vi "ShapeDetect_Setting_UI.vi"(8 "error in (no error)":errorcluster, 10 "ParameterIn":string, 11 "Vision_Image":T8(plugin-control)) -> (0 "error out":errorcluster, 1 "Cancel?":bool, 3 "ParameterOut":string)   [LabVIEW 2019]
uses:
  Controls/_UI Command Cluster/ShapeDetect_UICommand.ctl
  <vilib>/Utility/miscctls.llb/LVPointTypeDef.ctl
  Controls/V_Analysis_Type.ctl
  Controls/ShapeDectect/Analysis_ShapeDectect_Parameter.ctl
  Controls/Analysis_Setting.ctl
  <vilib>/vision/Image Controls.llb/IMAQ Image.ctl
  bd2e2234-6d1e-4fcc-8dd9-21a115e7fd9b.vi
  bb507319-f4b5-469f-81a6-a6debf547fbf.vi
  52026581-d36c-43e1-9bb6-5096a44cea8b.vi
  <vilib>/JDP Science/JSONtext/JSON text to Variant.vi
  <vilib>/JDP Science/JSONtext/Variant to JSON Text.vi
  <vilib>/vision/NI_Vision_Development_Module.lvlib
panel:
  in  "Show Curve":bool
  out "Message":string
  in  "Tab":enum32{"Curve", "Shape", "Setting", "Result"}(tab)
  in  "Curve Extraction":T1={"Extraction Mode"=0, "Edge Threshold"=75, "Edge Filter Size"=1, "Min Length"=25, "Row Search Step Size"=15, "Column Search Step Size"=15, "Max Endpoint Gap"=10, "Closed"=FALSE, "Subpixel"=FALSE} {"Edge Filter Size" items=["Fine", "Normal", "Contour Tracing"]; "Edge Threshold" min=0 max=255 step=1; "Extraction Mode" items=["Normal", "Uniform Regions"]}
  in  "Shape Type":T2(ring)
  out "DecriptroTab":T3(tab)
  in  "Circle Descriptor":T4={"Min Radius"=10.0, "Max Radius"=100.0, "Min"=10.0, "Max"=100.0} {"Max" min=10.0 max=100.0 step=1.0; "Min" min=3.0 max=10.0 step=1.0; "Min Radius" min=3.0 max=200.0 step=1.0; "Max Radius" min=10.0 step=1.0}
  in  "Ellipse Descriptor":T5={"Min Major Radius"=10.0, "Max Major Radius"=100.0, "Min Minor Radius"=10.0, "Max Minor Radius"=100.0} {"Max Major Radius" min=10.0 max=5000.0; "Min Major Radius" min=3.0 max=100.0 step=1.0; "Min Minor Radius" min=3.0 max=100.0 step=1.0; "Max Minor Radius" min=10.0 max=5000.0 step=1.0}
  in  "Line Descriptor":T6={"Min Length"=10.0, "Max Length"=100.0, "Min"=10.0, "Max"=100.0} {"Max" min=3.0 step=1.0; "Min" min=3.0 step=1.0; "Min Length" min=3.0 max=100.0 step=1.0; "Max Length" min=10.0 step=1.0}
  in  "Rectangle Descriptor":T7={"Min Height"=10.0, "Max Height"=100.0, "Min Width"=10.0, "Max Width"=100.0} {"Max Width" min=10.0 max=5000.0 step=1.0; "Min Width" min=3.0 max=100.0 step=1.0; "Min Height" min=3.0 max=100.0 step=1.0; "Max Height" min=10.0 max=5000.0 step=1.0}
  in  "Score":dbl=800.0 min=0.0 max=1000.0 step=1.0
  in  "Number to Detect":i32=1 min=1 step=1
  out "Result":string[][](table)
  in  "ReadImage":bool
  in  "Cancel":bool
  in  "OK":bool
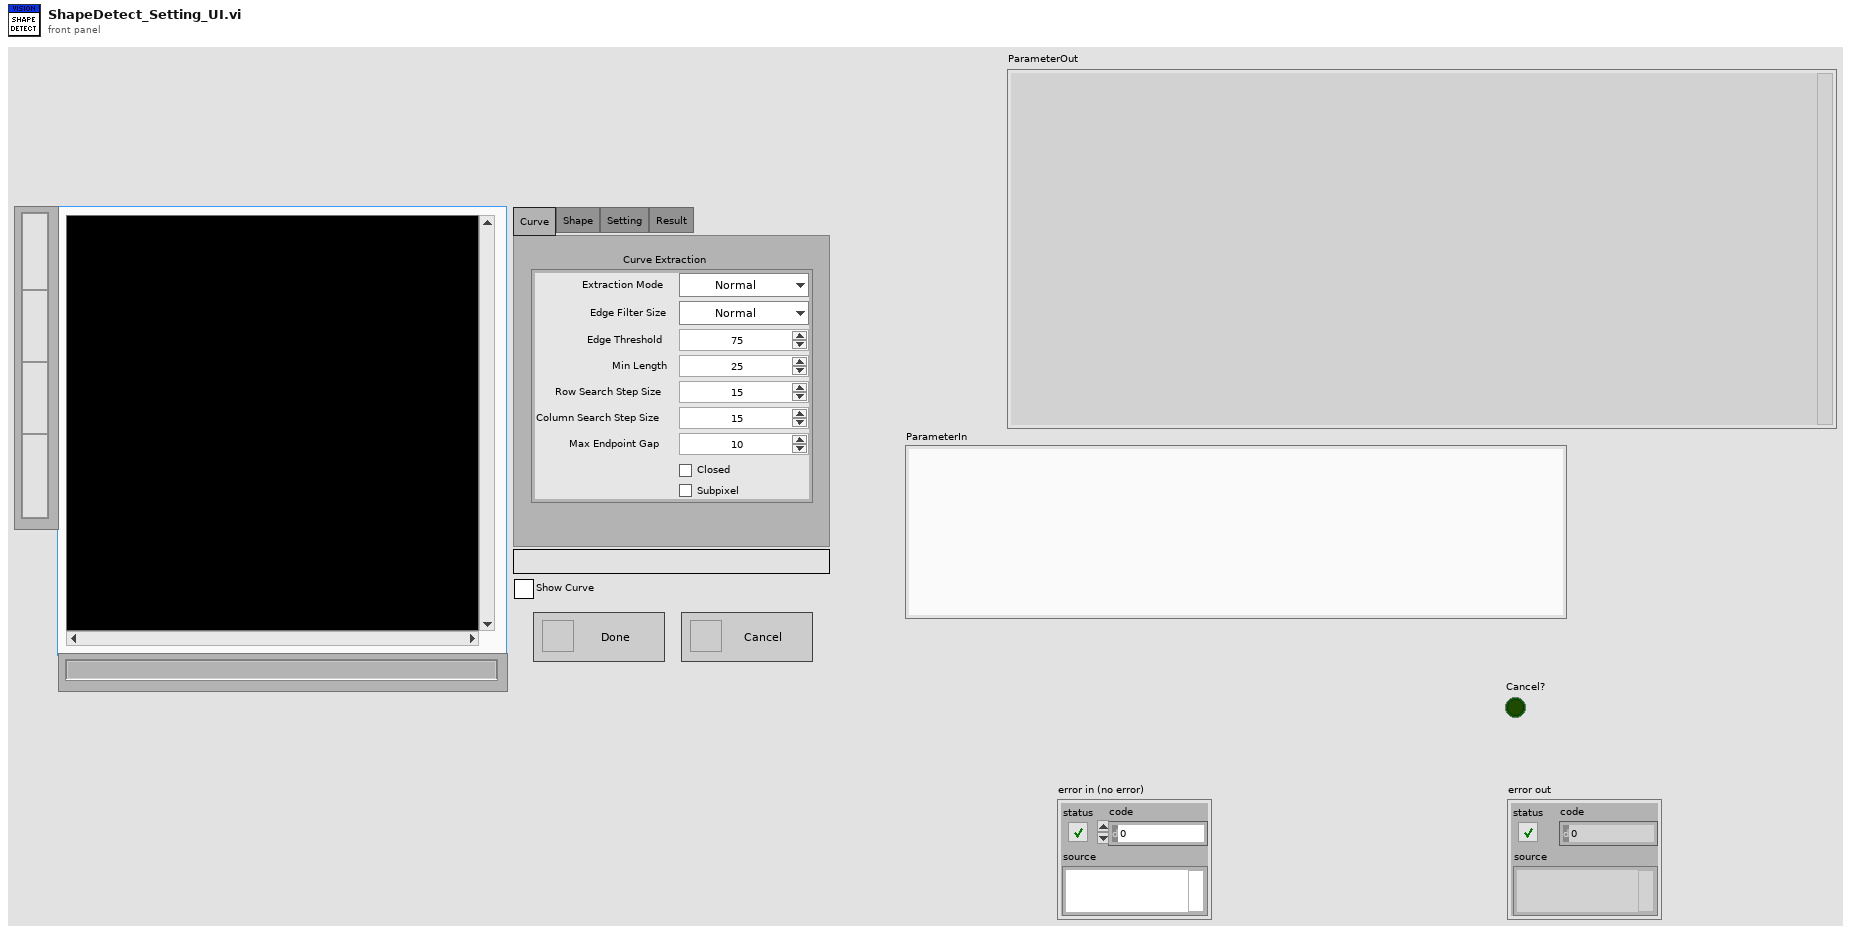
[diagram p1: front panel]
types:
  T1 = cluster{"Extraction Mode":u32, "Edge Threshold":i32, "Edge Filter Size":u32, "Min Length":i32, "Row Search Step Size":i32, "Column Search Step Size":i32, "Max Endpoint Gap":i32, "Closed":bool, "Subpixel":bool}
  T2 = enum16{"Circles", "Ellipses", "Lines", "Rectangles"}
  T3 = enum32{"Circles", "Ellipses", "Lines", "Rectangles"}
  T4 = cluster{"Min Radius":dbl, "Max Radius":dbl, "Min":dbl, "Max":dbl}
  T5 = cluster{"Min Major Radius":dbl, "Max Major Radius":dbl, "Min Minor Radius":dbl, "Max Minor Radius":dbl}
  T6 = cluster{"Min Length":dbl, "Max Length":dbl, "Min":dbl, "Max":dbl}
  T7 = cluster{"Min Height":dbl, "Max Height":dbl, "Min Width":dbl, "Max Width":dbl}
  T8 = typedef "IMAQ Image.ctl" = refnum<image>
  T9 = typedef "LVPointTypeDef.ctl" = cluster{"Horizontal":i16, "Vertical":i16}
  T10 = typedef "ShapeDetect_UICommand.ctl" = cluster{"Message":enum16{"Initialize", "InitializeUI", "CheckDescriptor", "RunAlgorithm", "Done", "Cancel", "Exit"}, "Data":variant}
  T11 = typedef "V_Analysis_Type.ctl" = enum16{"None", "C_Color Pattern Matching", "G_PatternMatching", "G_ShapeDectect", "G_GeometricMatch", "B_Area Check"}
  T12 = typedef "Analysis_ShapeDectect_Parameter.ctl" = cluster{"Enum_ShapeType":enum16{"Circles", "Ellipses", "Lines", "Rectangles"}, "MaxParticle":i32, "Descriptor":cluster{"Set 1":dbl, "Set 2":dbl, "Set 3":dbl, "Set 4":dbl}, "Match Options":cluster{"Rotation":bool, "Scale":bool, "Occlusion":bool, "Range Settings":cluster{"Match Constraints":u32, "Min":dbl, "Max":dbl}[]}, "Curve Parameters":cluster{"Extraction Mode":u32, "Edge Threshold":i32, "Edge Filter Size":u32, "Min Length":i32, "Row Search Step Size":i32, "Col Search Step Size":i32, "Max Endpoint Gap":i32, "Closed":bool, "Subpixel":bool}, " score":dbl}
  T13 = cluster{"Rotation":bool, "Scale":bool, "Occlusion":bool, "Range Settings":cluster{"Match Constraints":u32, "Min":dbl, "Max":dbl}[]}
  T14 = cluster{"Global Rectangle":i32[], "Contours":cluster{"ID":enum32{"External", "Internal"}, "Type":u32, "Coordinates":i32[]}[]}
  T15 = typedef "Analysis_Setting.ctl" = cluster{"PreProcess":T11, "Parameter":string}
  T16 = enum16{"Initialize", "InitializeUI", "CheckDescriptor", "RunAlgorithm", "Done", "Cancel", "Exit"}
  T17 = typedef "Image Type" = u32
  T18 = cluster{"Set 1":dbl, "Set 2":dbl, "Set 3":dbl, "Set 4":dbl}
  T19 = cluster{"Extraction Mode":u32, "Edge Threshold":i32, "Edge Filter Size":u32, "Min Length":i32, "Row Search Step Size":i32, "Col Search Step Size":i32, "Max Endpoint Gap":i32, "Closed":bool, "Subpixel":bool}
  T20 = typedef "IMAQ ExtractCurvesCurve.ctl" = cluster{"Points":cluster{"X":dbl, "Y":dbl}[], "Closed?":bool, "Curve Length":dbl, "Min Edge Strength":dbl, "Max Edge Strength":dbl, "Average Edge Strength":dbl}
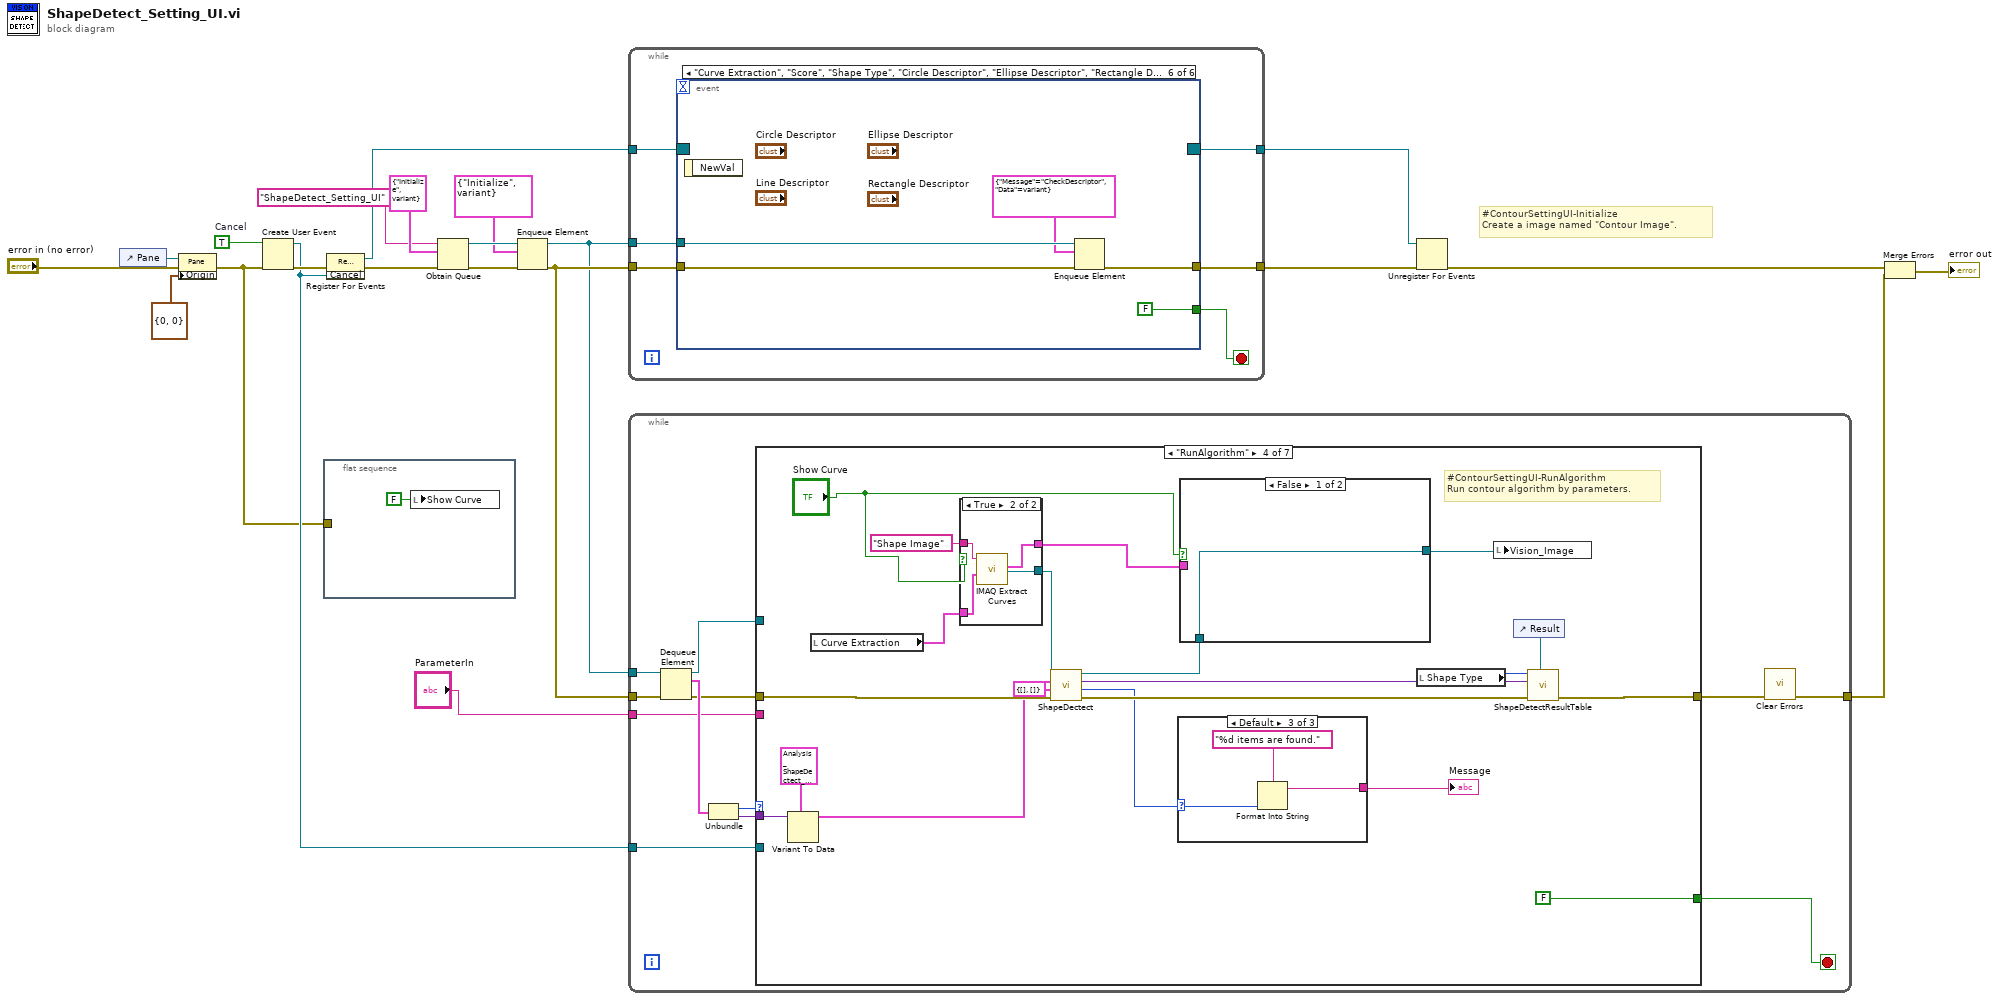
[diagram p0: block diagram]
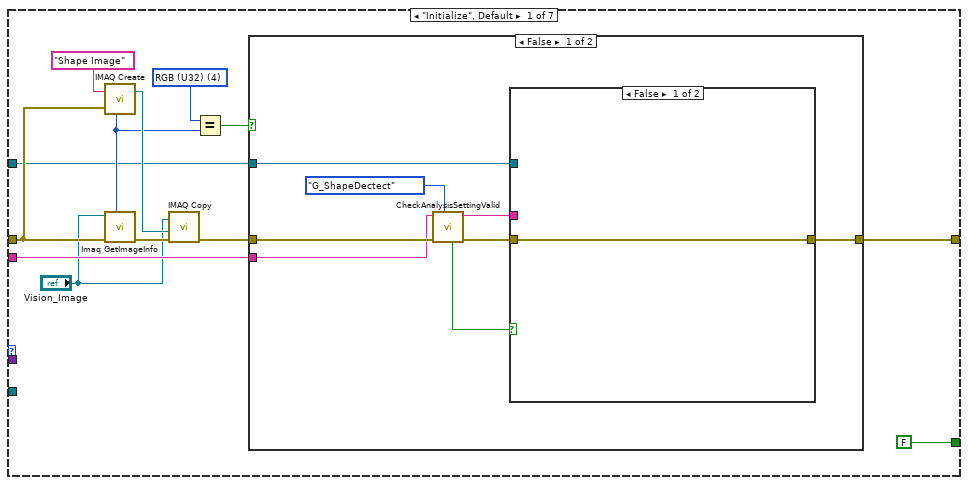
[diagram p2: hidden frame]
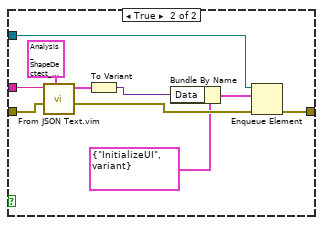
[diagram p3: hidden frame]
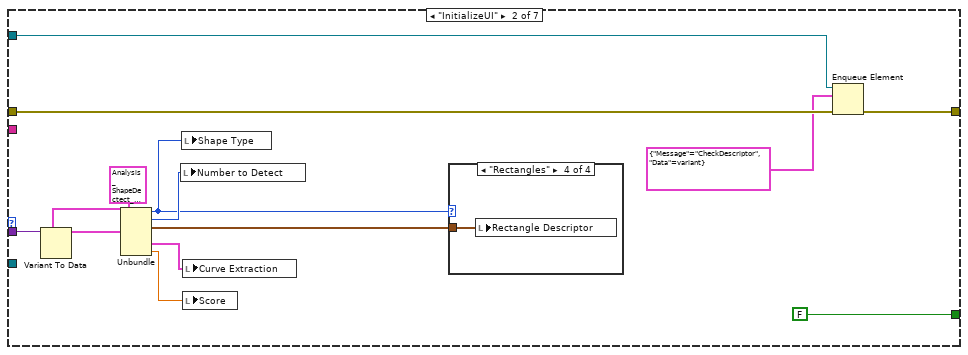
[diagram p5: hidden frame]
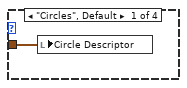
[diagram p6: hidden frame]
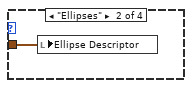
[diagram p7: hidden frame]
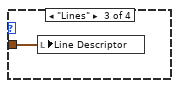
[diagram p8: hidden frame]
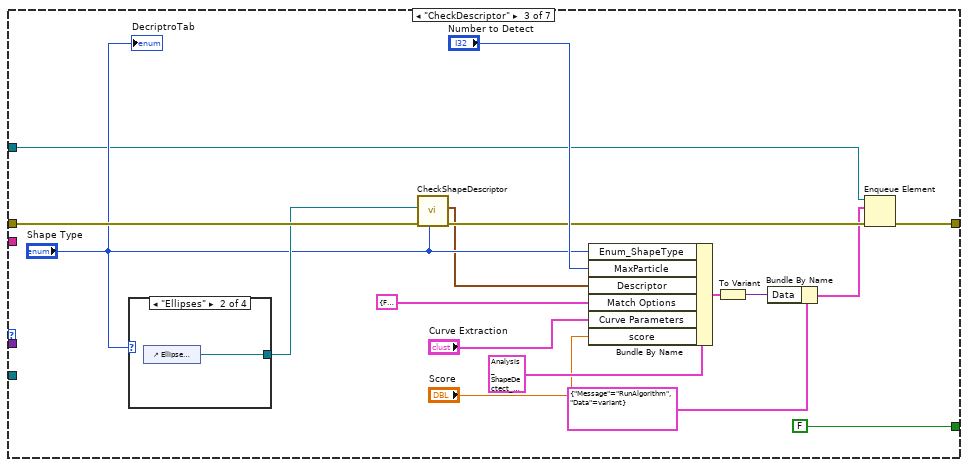
[diagram p9: hidden frame]
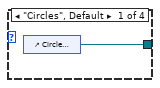
[diagram p10: hidden frame]
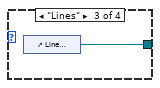
[diagram p11: hidden frame]
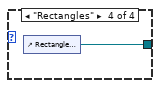
[diagram p12: hidden frame]
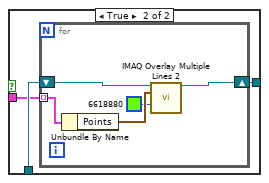
[diagram p13: hidden frame]
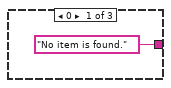
[diagram p15: hidden frame]
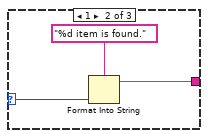
[diagram p16: hidden frame]
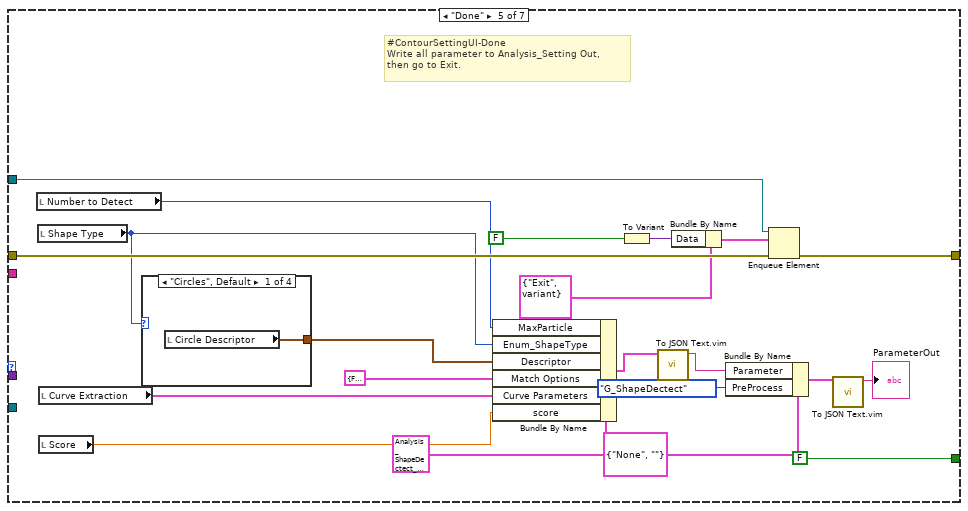
[diagram p17: hidden frame]
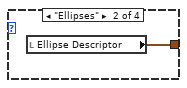
[diagram p18: hidden frame]
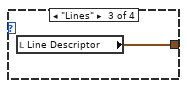
[diagram p19: hidden frame]
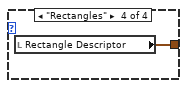
[diagram p20: hidden frame]
diagram:
  w16 = TRUE  # Cancel
  # "#ContourSettingUI-Initialize\nCreate a image named \"Contour Image\"."
  n1 = control-ref of="Pane"() -> (w9:refnum<vi>)
  n2 = property class="Pane"(reference=w9, error in="error in (no error)", "Origin"=T9 {"Horizontal"=0, "Vertical"=0}) -> (error out=w1:errorcluster)  [unwired: 1 out]
  n3 = Create User Event(user event datatype=w16, error in=w1) -> (user event=w10:refnum<user-event>, error out=w17:errorcluster)
  n4 = flat-sequence {
    tunnel: w1 -> [_]
    frame #0 {
      n5 = local write "Show Curve"(FALSE ("Show Curve")) -> ()
    }
  }
  n6 = register-events(error in=w17, w10) -> (reference out=w15:refnum<event-registration>, error out=w18:errorcluster)  [unwired: 1 in]
  n7 = Obtain Queue(name (unnamed)="ShapeDetect_Setting_UI", element data type=T10 {"Message"=enum."Initialize", "Data"=variant} ("_UICommand"), error in (no error)=w18) -> (queue out=w21:refnum<queue>, error out=w22:errorcluster)  [unwired: 2 in, 1 out]
  n8 = Enqueue Element(queue=w21, element=T10 {"Message"=enum."Initialize", "Data"=variant} ("_UICommand"), error in (no error)=w22) -> (queue out=w19:refnum<queue>, error out=w20:errorcluster)  [unwired: 1 in, 1 out]
  n9 = while {
    tunnel: w19 -> [w29]
    tunnel: w20 -> [w28]
    tunnel: w15 -> [w27]
    tunnel: [w26] -> w14
    tunnel: [w25] -> w13
    stop <- w24 stop-if-true
    n10 = event shown="[5] \"Curve Extraction\", \"Score\", \"Shape Type\", \"Circle Descriptor\", \"Ellipse Descriptor\", \"Rectangle Descriptor\", \"Line Descriptor\", \"Number to Detect\", \"Show Curve\": Value Change" {
      selector: w27 -> [_ _ _ _ _ _]
      dyn-events: [_ _ _ _ _ _] -> w26
      timeout: _ -> [_ _ _ _ _ _]
      tunnel: w29 -> [_ w34 w39 w46 _ w62]
      tunnel: w28 -> [w31 w35 w41 w45 w51 w61]
      tunnel: [w31 w36 w40 w44 w50 w60] -> w25
      tunnel: [FALSE TRUE TRUE TRUE FALSE FALSE] -> w24
      event Timeout {
        n11 = event-data() -> ()  [unwired: 1 in, 1 out]
      }
      event "OK": Value Change {
        n12 = event-data() -> ()  [unwired: 1 in, 1 out]
        n13 = Enqueue Element(queue=w34, element=T10 {"Message"=enum."Done", "Data"=variant} ("_UICommand"), error in (no error)=w35) -> (error out=w36:errorcluster)  [unwired: 1 in, 2 out]
      }
      event "Cancel": Value Change {
        n14 = event-data() -> ()  [unwired: 1 in, 1 out]
        n15 = Enqueue Element(queue=w39, element=T10 {"Message"=enum."Cancel", "Data"=variant} ("_UICommand"), error in (no error)=w41) -> (error out=w40:errorcluster)  [unwired: 1 in, 2 out]
      }
      event User Event {
        n16 = event-data() -> ()  [unwired: 1 in, 1 out]
        n17 = Enqueue Element(queue=w46, element=T10 {"Message"=enum."Cancel", "Data"=variant} ("_UICommand"), error in (no error)=w45) -> (error out=w44:errorcluster)  [unwired: 1 in, 2 out]
      }
      event "ReadImage": Value Change {
        n18 = event-data() -> ()  [unwired: 1 in, 1 out]
        n19 = call "IMAQ Load Image Dialog"() -> ("Cancelled?"=w48:bool, "Path"=w47:path)  [unwired: 9 in, 1 out]
        n20 = case shown="True" w48 {
          tunnel: w51 -> [w56 w57]
          tunnel: [w55 w57] -> w50
          tunnel: w47 -> [w53 _]
          frame False {
            n21 = call "IMAQ ReadFile"("File Path"=w53, "error in (no error)"=w56, "Image"="Shape Image" ("Image Name")) -> ("error out"=w55:errorcluster, "Image Out"=w52:T8)  [unwired: 4 in, 3 out]
            n22 = local write "Vision_Image"(w52) -> ()
          }
          frame True {
          }
        }
      }
      event "Curve Extraction", "Score", "Shape Type", "Circle Descriptor", "Ellipse Descriptor", "Rectangle Descriptor", "Line Descriptor", "Number to Detect", "Show Curve": Value Change {
        n23 = event-data() -> ()  [unwired: 1 in, 1 out]
        n24 = Enqueue Element(queue=w62, element=T10 {"Message"=enum."CheckDescriptor", "Data"=variant} ("_UICommand"), error in (no error)=w61) -> (error out=w60:errorcluster)  [unwired: 1 in, 2 out]
      }
    }
  }
  n25 = while {
    tunnel: w20 -> [w74]
    tunnel: w19 -> [w73]
    tunnel: w10 -> [w67]
    tunnel: [w65] -> w4
    tunnel: "ParameterIn" -> [w63]
    stop <- w66 stop-if-true
    n26 = Dequeue Element(queue=w73, error in (no error)=w74) -> (queue out=w71:refnum<queue>, element=w72:T10, error out=w69:errorcluster)  [unwired: 1 in, 1 out]
    n27 = Unbundle(w72) -> ("Message"=w70:T16, "Data"=w68:variant)
    n28 = case shown="\"RunAlgorithm\"" w70 {
      tunnel: w71 -> [w78 w111 w132 _ w204 w215 w223]
      tunnel: w69 -> [w84 w112 w140 w163 w206 w217 w229]
      tunnel: w68 -> [_ w119 _ w157 _ _ w222]
      tunnel: [FALSE FALSE FALSE FALSE FALSE FALSE TRUE] -> w66
      tunnel: w67 -> [_ _ _ _ _ _ w227]
      tunnel: [w77 w110 w134 w160 w205 w216 w224] -> w64
      tunnel: w63 -> [w76 _ _ _ _ _ _]
      frame "Initialize", Default {
        w83 = T17 4 items=["Grayscale (U8)", "Grayscale (I16)", "Grayscale (SGL)", "Complex (CSG)", "RGB (U32)", "HSL (U32)", "RGB (U64)", "Grayscale (U16)"] ("x")
        n29 = call "Imaq GetImageInfo"("error in (no error)"=w84, "Image"="Vision_Image") -> ("error out"=w85:errorcluster, "Image Type"=w81:T17)  [unwired: 2 in, 6 out]
        n30 = call "IMAQ Create"("Image Name"="Shape Image", "Image Type"=w81, "error in (no error)"=w84) -> ("New Image"=w82:T8)  [unwired: 2 in, 1 out]
        n31 = call "IMAQ Copy"("error in (no error)"=w85, "Image Dst"=w82, "Image Src"="Vision_Image") -> ("error out"=w79:errorcluster)  [unwired: 3 in, 1 out]
        n32 = Equal?(x=w83, y=w81) -> (x = y?=w80:bool)
        n33 = case shown="False" w80 {
          tunnel: w79 -> [w95 w107]
          tunnel: w78 -> [w89 _]
          tunnel: [w91 w107] -> w77
          tunnel: w76 -> [w88 _]
          frame False {
            n34 = call "CheckAnalysisSettingValid.vi"("Analysis_Type"=V_Analysis_Type."G_ShapeDectect", "error in (no error)"=w95, "ParameterIn"=w88) -> ("error out"=w93:errorcluster, "ParameterOut"=w92:string, "Valid"=w94:bool)  [unwired: 6 in]
            n35 = case shown="False" w94 {
              tunnel: w93 -> [w96 w97]
              tunnel: w92 -> [_ w106]
              tunnel: w89 -> [_ w102]
              tunnel: [w96 w98] -> w91
              frame False {
              }
              frame True {
                n36 = call "From JSON Text.vim"("Data Type and Default Value"=T12 {"Enum_ShapeType"=enum."Circles", "MaxParticle"=1, "Descriptor"={"Set 1"=10.0, "Set 2"=100.0, "Set 3"=200.0, "Set 4"=10.0}, "Match Options"={"Rotation"=TRUE, "Scale"=FALSE, "Occlusion"=FALSE, "Range Settings"=[{"Match Constraints"=0, "Min"=0.0, "Max"=360.0}]}, "Curve Parameters"={"Extraction Mode"=0, "Edge Threshold"=75, "Edge Filter Size"=1, "Min Length"=25, "Row Search Step Size"=15, "Col Search Step Size"=15, "Max Endpoint Gap"=10, "Closed"=FALSE, "Subpixel"=FALSE}, " score"=500.0} ("ShapeDetectParameter"), "error in (no error)"=w97, "JSON"=w106) -> ("error out"=w103:errorcluster, "Data out"=w104:T12)  [unwired: 7 in]
                n37 = To Variant(anything=w104) -> (Variant=w100:variant)
                n38 = Bundle By Name(cluster=T10 {"Message"=enum."InitializeUI", "Data"=variant} ("_UICommand"), "Data"=w100) -> (w99:T10)
                n39 = Enqueue Element(queue=w102, element=w99, error in (no error)=w103) -> (error out=w98:errorcluster)  [unwired: 1 in, 2 out]
              }
            }
          }
          frame True {
          }
        }
      }
      frame "InitializeUI" {
        n40 = Variant To Data(type=T12 {"Enum_ShapeType"=enum."Circles", "MaxParticle"=1, "Descriptor"={"Set 1"=10.0, "Set 2"=100.0, "Set 3"=200.0, "Set 4"=10.0}, "Match Options"={"Rotation"=TRUE, "Scale"=FALSE, "Occlusion"=FALSE, "Range Settings"=[{"Match Constraints"=0, "Min"=0.0, "Max"=360.0}]}, "Curve Parameters"={"Extraction Mode"=0, "Edge Threshold"=75, "Edge Filter Size"=1, "Min Length"=25, "Row Search Step Size"=15, "Col Search Step Size"=15, "Max Endpoint Gap"=10, "Closed"=FALSE, "Subpixel"=FALSE}, " score"=500.0} ("ShapeDetectParameter"), Variant=w119) -> (data=w109:T12)  [unwired: 1 in, 1 out]
        n41 = Unbundle(w109) -> ("Enum_ShapeType"=w115:T2, "MaxParticle"=w117:i32, "Descriptor"=w114:T18, "Curve Parameters"=w116:T19, "score"=w118:dbl)  [unwired: 1 out]
        n42 = local write "Number to Detect"(w117) -> ()
        n43 = local write "Shape Type"(w115) -> ()
        n44 = local write "Curve Extraction"(w116) -> ()
        n45 = local write "Score"(w118) -> ()
        n46 = case shown="\"Rectangles\"" w115 {
          tunnel: w114 -> [w121 w122 w123 w124]
          frame "Circles", Default {
            n47 = local write "Circle Descriptor"(w121) -> ()
          }
          frame "Ellipses" {
            n48 = local write "Ellipse Descriptor"(w122) -> ()
          }
          frame "Lines" {
            n49 = local write "Line Descriptor"(w123) -> ()
          }
          frame "Rectangles" {
            n50 = local write "Rectangle Descriptor"(w124) -> ()
          }
        }
        n51 = Enqueue Element(queue=w111, element=T10 {"Message"=enum."CheckDescriptor", "Data"=variant} ("_UICommand"), error in (no error)=w112) -> (error out=w110:errorcluster)  [unwired: 1 in, 2 out]
      }
      frame "CheckDescriptor" {
        n52 = case shown="\"Ellipses\"" "Shape Type" {
          tunnel: [w142 w143 w144 w145] -> w136
          frame "Circles", Default {
            n53 = control-ref of="Circle Descriptor"() -> (w142:refnum<vi>)
          }
          frame "Ellipses" {
            n54 = control-ref of="Ellipse Descriptor"() -> (w143:refnum<vi>)
          }
          frame "Lines" {
            n55 = control-ref of="Line Descriptor"() -> (w144:refnum<vi>)
          }
          frame "Rectangles" {
            n56 = control-ref of="Rectangle Descriptor"() -> (w145:refnum<vi>)
          }
        }
        n57 = call "CheckShapeDescriptor.vi"("Shape Type"="Shape Type", "error in (no error)"=w140, "Descriptor Ref"=w136) -> ("error out"=w133:errorcluster, "Descriptor"=w125:T18)  [unwired: 7 in]
        n58 = Bundle By Name(cluster=T12 {"Enum_ShapeType"=enum."Circles", "MaxParticle"=1, "Descriptor"={"Set 1"=10.0, "Set 2"=100.0, "Set 3"=200.0, "Set 4"=10.0}, "Match Options"={"Rotation"=TRUE, "Scale"=FALSE, "Occlusion"=FALSE, "Range Settings"=[{"Match Constraints"=0, "Min"=0.0, "Max"=360.0}]}, "Curve Parameters"={"Extraction Mode"=0, "Edge Threshold"=75, "Edge Filter Size"=1, "Min Length"=25, "Row Search Step Size"=15, "Col Search Step Size"=15, "Max Endpoint Gap"=10, "Closed"=FALSE, "Subpixel"=FALSE}, " score"=500.0} ("ShapeDetectParameter"), "Enum_ShapeType"="Shape Type", "MaxParticle"="Number to Detect", "Descriptor"=w125, "Match Options"=T13 {"Rotation"=FALSE, "Scale"=FALSE, "Occlusion"=FALSE, "Range Settings"=[]}, "Curve Parameters"="Curve Extraction", "score"="Score") -> (w130:T12)
        n59 = To Variant(anything=w130) -> (Variant=w129:variant)
        n60 = Bundle By Name(cluster=T10 {"Message"=enum."RunAlgorithm", "Data"=variant} ("_UICommand"), "Data"=w129) -> (w128:T10)
        n61 = Enqueue Element(queue=w132, element=w128, error in (no error)=w133) -> (error out=w134:errorcluster)  [unwired: 1 in, 2 out]
        "DecriptroTab" <- "Shape Type"
      }
      frame "RunAlgorithm" {
        # "#ContourSettingUI-RunAlgorithm\nRun contour algorithm by parameters."
        n62 = Variant To Data(type=T12 {"Enum_ShapeType"=enum."Circles", "MaxParticle"=1, "Descriptor"={"Set 1"=10.0, "Set 2"=100.0, "Set 3"=200.0, "Set 4"=10.0}, "Match Options"={"Rotation"=TRUE, "Scale"=FALSE, "Occlusion"=FALSE, "Range Settings"=[{"Match Constraints"=0, "Min"=0.0, "Max"=360.0}]}, "Curve Parameters"={"Extraction Mode"=0, "Edge Threshold"=75, "Edge Filter Size"=1, "Min Length"=25, "Row Search Step Size"=15, "Col Search Step Size"=15, "Max Endpoint Gap"=10, "Closed"=FALSE, "Subpixel"=FALSE}, " score"=500.0} ("ShapeDetectParameter"), Variant=w157) -> (data=w153:T12)  [unwired: 1 in, 1 out]
        n63 = local read "Curve Extraction"() -> (w150:T1)
        n64 = case shown="True" "Show Curve" {
          tunnel: [w175 w179] -> w152
          tunnel: "Shape Image" ("Image Name") -> [w175 w178]
          tunnel: w150 -> [_ w177]
          tunnel: [_ w176] -> w148
          frame False {
          }
          frame True {
            n65 = call "IMAQ Extract Curves"("Curve Parameters"=w177, "Image"=w178) -> ("Curves"=w176:T20[], "Image (dup)"=w179:T8)  [unwired: 7 in, 1 out]
          }
        }
        n66 = call "ShapeDectect.vi"("error in (no error)"=w163, "ROI Descriptor"=T14 {"Global Rectangle"=[], "Contours"=[]}, "SetParameter"=w153, "Image In"=w152) -> ("error out"=w162:errorcluster, "DectectItem"=w155:i32, "ResultOut"=w161:variant, "Image Out"=w164:T8)  [unwired: 4 in]
        n67 = case shown="Default" w155 {
          selector: w155 -> [_ w183 w186]
          tunnel: ["No item is found." w181 w184] -> w154
          frame 0 {
          }
          frame 1 {
            n68 = Format Into String(format string="%d item is found.", w183) -> (resulting string=w181:string)  [unwired: 2 in, 1 out]
          }
          frame Default {
            n69 = Format Into String(format string="%d items are found.", w186) -> (resulting string=w184:string)  [unwired: 2 in, 1 out]
          }
        }
        "Message" <- w154
        n70 = case shown="False" "Show Curve" {
          tunnel: w164 -> [w166 w169]
          tunnel: [w166 w168] -> w149
          tunnel: w148 -> [_ w167]
          frame False {
          }
          frame True {
            n71 = for {
              shift-right: [w173] -> w168
              shift-left: w169 -> [w174]
              tunnel: w167 -> [w172] mode=indexing
              n72 = Unbundle By Name(w172) -> ("Points"=w171:cluster{"X":dbl, "Y":dbl}[])
              n73 = call "IMAQ Overlay Multiple Lines 2"("Image"=w174, "Line End Points"=w171, "Color"=u32 6618880) -> ("Image Out"=w173:T8)  [unwired: 11 in, 1 out]
            }
          }
        }
        n74 = local read "Shape Type"() -> (w158:T2)
        n75 = local write "Vision_Image"(w149) -> ()
        n76 = control-ref of="Result"() -> (w159:refnum<vi>)
        n77 = call "ShapeDetectResultTable.vi"("Table"=w159, "error in (no error)"=w162, "Result"=w161, "Shape Type"=w158) -> ("error out"=w160:errorcluster)  [unwired: 7 in]
      }
      frame "Done" {
        # "#ContourSettingUI-Done\nWrite all parameter to Analysis_Setting Out,\nthen go to Exit."
        n78 = local read "Number to Detect"() -> (w197:i32)
        n79 = local read "Shape Type"() -> (w195:T2)
        n80 = local read "Curve Extraction"() -> (w194:T1)
        n81 = local read "Score"() -> (w193:dbl)
        n82 = case shown="\"Circles\", Default" w195 {
          tunnel: [w208 w209 w210 w211] -> w196
          frame "Circles", Default {
            n83 = local read "Circle Descriptor"() -> (w208:T4)
          }
          frame "Ellipses" {
            n84 = local read "Ellipse Descriptor"() -> (w209:T5)
          }
          frame "Lines" {
            n85 = local read "Line Descriptor"() -> (w210:T6)
          }
          frame "Rectangles" {
            n86 = local read "Rectangle Descriptor"() -> (w211:T7)
          }
        }
        n87 = Bundle By Name(cluster=T12 {"Enum_ShapeType"=enum."Circles", "MaxParticle"=1, "Descriptor"={"Set 1"=10.0, "Set 2"=100.0, "Set 3"=200.0, "Set 4"=10.0}, "Match Options"={"Rotation"=TRUE, "Scale"=FALSE, "Occlusion"=FALSE, "Range Settings"=[{"Match Constraints"=0, "Min"=0.0, "Max"=360.0}]}, "Curve Parameters"={"Extraction Mode"=0, "Edge Threshold"=75, "Edge Filter Size"=1, "Min Length"=25, "Row Search Step Size"=15, "Col Search Step Size"=15, "Max Endpoint Gap"=10, "Closed"=FALSE, "Subpixel"=FALSE}, " score"=500.0} ("ShapeDetectParameter"), "MaxParticle"=w197, "Enum_ShapeType"=w195, "Descriptor"=w196, "Match Options"=T13 {"Rotation"=FALSE, "Scale"=FALSE, "Occlusion"=FALSE, "Range Settings"=[]}, "Curve Parameters"=w194, "score"=w193) -> (w190:T12)
        n88 = To Variant(anything=FALSE) -> (Variant=w202:variant)
        n89 = call "To JSON Text.vim"("Anything"=w190) -> ("<JSON>"=w191:string)  [unwired: 9 in, 1 out]
        n90 = Bundle By Name(cluster=T10 {"Message"=enum."Exit", "Data"=variant} ("_UICommand"), "Data"=w202) -> (w201:T10)
        n91 = Bundle By Name(cluster=T15 {"PreProcess"=enum."None", "Parameter"=""} ("Analysis_Setting Out"), "Parameter"=w191, "PreProcess"=V_Analysis_Type."G_ShapeDectect") -> (w189:T15)
        n92 = Enqueue Element(queue=w204, element=w201, error in (no error)=w206) -> (error out=w205:errorcluster)  [unwired: 1 in, 2 out]
        n93 = call "To JSON Text.vim"("Anything"=w189) -> ("<JSON>"=→"ParameterOut":string)  [unwired: 9 in, 1 out]
      }
      frame "Cancel" {
        # "#ContourSettingUI-Cancel\nDo nothing, then go to Exit."
        n94 = To Variant(anything=TRUE) -> (Variant=w212:variant)
        n95 = Bundle By Name(cluster=T10 {"Message"=enum."Exit", "Data"=variant} ("_UICommand"), "Data"=w212) -> (w214:T10)
        n96 = Enqueue Element(queue=w215, element=w214, error in (no error)=w217) -> (error out=w216:errorcluster)  [unwired: 1 in, 2 out]
      }
      frame "Exit" {
        (unwired) T8 refnum ("Vision_Image")
        # "#ContourSettingUI-Exit\nRealease Queue, stop the loop, then close the window."
        n97 = Variant To Data(type=TRUE ("Cancel?"), Variant=w222) -> (data=→"Cancel?":bool)  [unwired: 1 in, 1 out]
        n98 = Release Queue(queue=w223, error in (no error)=w229) -> (error out=w225:errorcluster)  [unwired: 1 in, 2 out]
        n99 = Destroy User Event(user event=w227) -> ()  [unwired: 1 in, 1 out]
        n100 = call "IMAQ Dispose"("Image"="Shape Image" ("Image Name"), "error in (no error)"=w225) -> ("error out"=w224:errorcluster)  [unwired: 4 in]
      }
    }
    n101 = call <vilib>:"Clear Errors.vi"("error in (no error)"=w64) -> ("error out"=w65:errorcluster)  [unwired: 5 in, 1 out]
  }
  n102 = Unregister For Events(event registration refnum=w14, error in=w13) -> (error out=w5:errorcluster)
  n103 = Merge Errors(w5, w4) -> (→"error out":errorcluster)
